vi "Lookup Condition Type.vi"(8 "error in (no error)":errorcluster, 10 "Condition Type":string) -> (0 "error out":errorcluster, 2 "Condition":refnum<class "Condition Config.lvclass">)   [LabVIEW 2020, in "VolatusSeqConfig.lvlib"]
uses:
  VolatusSeqConfig.lvlib
  Condition Config/Condition Config.lvclass
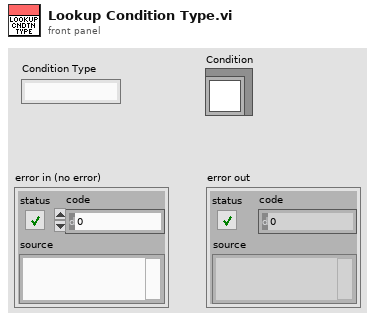
[diagram p1: front panel]
types:
  T1 = map{string, refnum<class "Condition Config.lvclass">}
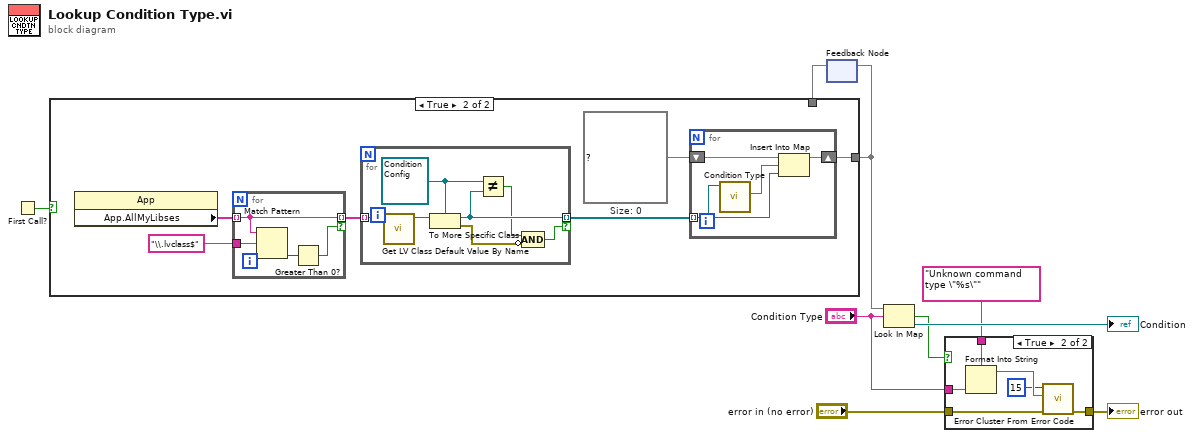
[diagram p0: block diagram]
diagram:
  n1 = First Call?() -> (First Call?: T/F=w9:bool)
  n2 = feedback #1() -> (w8:T1)  [unwired: 1 in]
  n3 = case shown="True" w9 {
    tunnel: [w10 w11] -> w7
    tunnel: w8 -> [w10 _]
    frame False {
    }
    frame True {
      w13 = T1 {}  # Size: 0
      n4 = property class="App"() -> ("App.AllMyLibses"=w16:string[])  [unwired: 2 in, 2 out]
      n5 = for {
        tunnel: w16 -> [w29] mode=indexing
        tunnel: "\\.lvclass$" -> [w31]
        tunnel: [w29] -> w14 mode=indexing if=w28
        n6 = Match Pattern(string=w29, regular expression=w31) -> (offset past match=w30:i32)  [unwired: 1 in, 3 out]
        n7 = Greater Than 0?(x=w30) -> (x > 0?=w28:bool)
      }
      n8 = for {
        tunnel: w14 -> [w27] mode=indexing
        tunnel: [w24] -> w12 mode=indexing if=w21
        w25 = refnum<class "Condition Config.lvclass"> refnum ("VolatusSeqConfig.lvlib:Condition Config.lvclass")
        n9 = call <vilib>:"Get LV Class Default Value By Name.vi"("class name"=w27) -> ("object"=w26:refnum<class>)  [unwired: 9 in, 1 out]
        n10 = To More Specific Class(target class=w25, reference=w26) -> (specific class reference=w24:refnum<class "Condition Config.lvclass">, error out=w22:errorcluster)  [unwired: 1 in]
        n11 = Not Equal?(x=w25, y=w24) -> (x != y?=w23:bool)
        n12 = Compound Arithmetic op=AND(w23, invert w22) -> (w21:bool)
      }
      n13 = for {
        shift-right: [w18] -> w11
        shift-left: w13 -> [w20]
        tunnel: w12 -> [w17] mode=indexing
        n14 = call-dynamic "Condition Type.vi"("Condition Config in"=w17) -> ("Condition Type"=w19:string)  [unwired: 10 in]
        n15 = Insert Into Map(map in=w20, key=w19, value=w17) -> (map out=w18:T1)  [unwired: 2 out]
      }
    }
  }
  n16 = feedback-in #1(w7) -> ()
  n17 = Look In Map(map=w7, key="Condition Type") -> (key not found?=w5:bool, value=→"Condition":refnum<class "Condition Config.lvclass">)  [unwired: 1 in]
  n18 = case shown="True" w5 {
    tunnel: "Unknown command type \"%s\"" -> [_ w38]
    tunnel: "Condition Type" -> [_ w37]
    tunnel: [w32 w34] -> w2
    tunnel: "error in (no error)" -> [w32 w33]
    frame False {
    }
    frame True {
      n19 = Format Into String(format string=w38, w37) -> (resulting string=w36:string)  [unwired: 2 in, 1 out]
      n20 = call <vilib>:"Error Cluster From Error Code.vi"("error in (no error)"=w33, "error message (\"\")"=w36, "error code (0)"=15) -> ("error out"=w34:errorcluster)  [unwired: 6 in]
    }
  }
  "error out" <- w2
